vi "Untitled 13 (SubVI)original.vi"(0 "time":dbl[](array[numeric]), 5 "acceleration":dbl[](array[numeric])) -> (1 "Frequency Interval: delta(f)":dbl, 2 "Spectrum plot":cluster{i32, dbl, "spectrum out":dbl[]}(graph), 3 "size(s)":i32, 4 "all rows":dbl[](array[numeric]), 6 "df (Hz)":dbl, 8 "Array":dbl[](array[numeric]), 10 "xf (frequency)":dbl[](array[numeric]), 12 "ploted signal from each selected frequency":dbl[][](graph), 14 "phase 2":dbl[](array[numeric]), 15 "magnitude 2":dbl[](array[numeric]))   [LabVIEW 2020]
uses:
  <vilib>/Analysis/2dsp.llb/Real FFT.vi
  <vilib>/Analysis/NI_AALPro.lvlib
  <vilib>/rvi/Analysis/host/Public/NI_FpgaMspHost.lvlib
  <vilib>/ptbypt/NI_PtbyPt.lvlib
panel:
  out "XY Graph":cluster{dbl[], dbl[]}(graph)
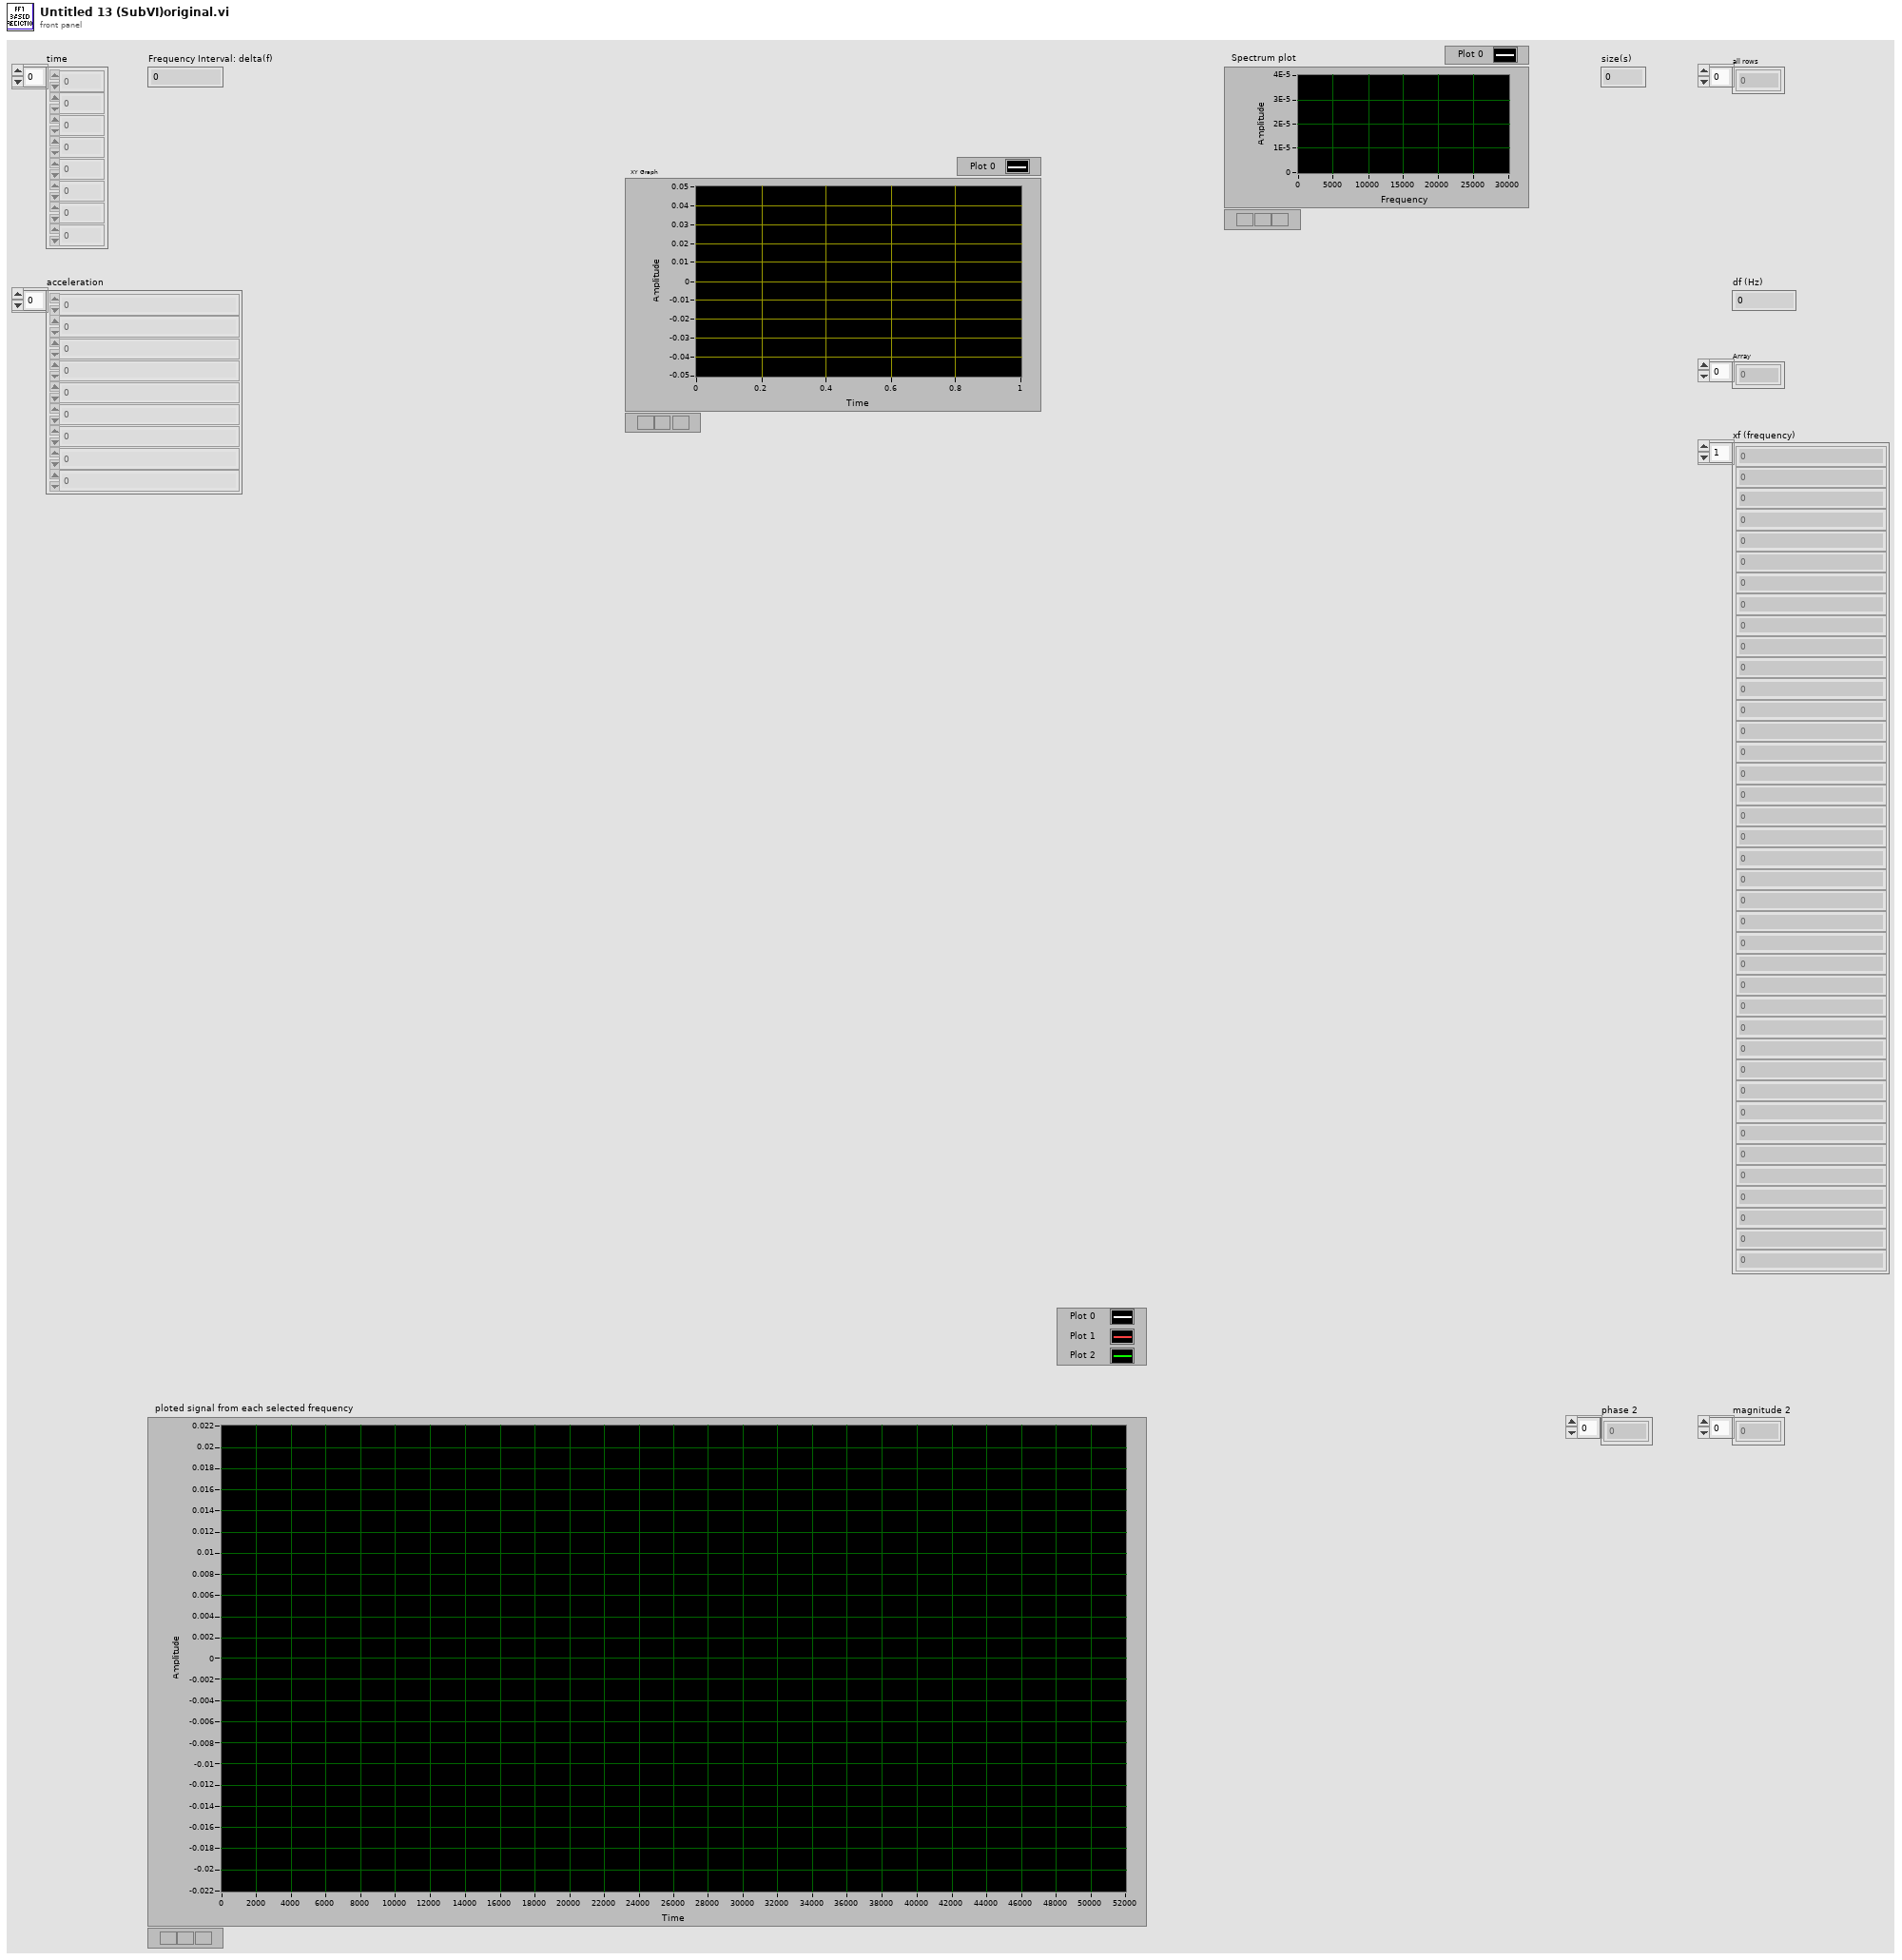
[diagram p1: front panel]
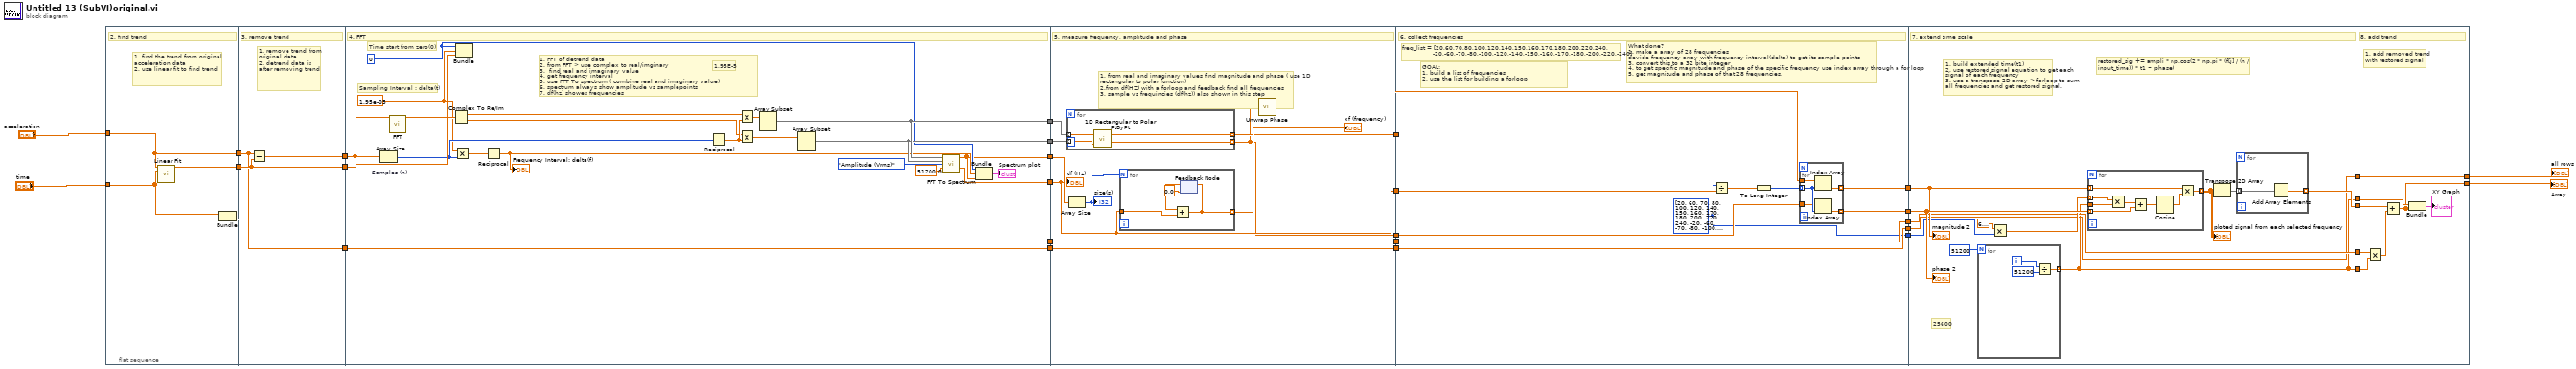
[diagram p0: block diagram]
diagram:
  n1 = flat-sequence {
    tunnel: [w33] -> w30
    tunnel: [w32] -> w29
    tunnel: "acceleration" -> [w32]
    tunnel: "time" -> [w31]
    tunnel: w30 -> [w35]
    tunnel: w29 -> [w34]
    tunnel: [w36] -> w28
    tunnel: [w35] -> w27
    tunnel: [w34] -> w26
    tunnel: w28 -> [w51]
    tunnel: [w50] -> w25
    tunnel: [w49] -> w24
    tunnel: [w42] -> w23
    tunnel: [w38] -> w22
    tunnel: [w37] -> w21
    tunnel: w27 -> [w37]
    tunnel: w26 -> [w40]
    tunnel: [w40] -> w20
    tunnel: w25 -> [w67]
    tunnel: w24 -> [w66]
    tunnel: w23 -> [w62]
    tunnel: w22 -> [w64]
    tunnel: [w62] -> w19
    tunnel: [w61] -> w18
    tunnel: [w60] -> w17
    tunnel: [w59] -> w16
    tunnel: w21 -> [w59]
    tunnel: w20 -> [w58]
    tunnel: [w58] -> w15
    tunnel: w19 -> [w77]
    tunnel: [w83] -> w14
    tunnel: w18 -> [w82]
    tunnel: w17 -> [w81]
    tunnel: [w80] -> w13
    tunnel: [w76] -> w12
    tunnel: [w79] -> w11
    tunnel: w16 -> [w79]
    tunnel: w15 -> [w78]
    tunnel: [w78] -> w10
    tunnel: w14 -> [w100]
    tunnel: w13 -> [w101]
    tunnel: w12 -> [w96]
    tunnel: [w94] -> w9
    tunnel: [w93] -> w8
    tunnel: w11 -> [w93]
    tunnel: [w92] -> w7
    tunnel: [w92] -> w6
    tunnel: w10 -> [w91]
    tunnel: [w91] -> w5
    tunnel: w9 -> [w123]
    tunnel: w8 -> [w121]
    tunnel: w7 -> [w122]
    tunnel: w6 -> [w120]
    tunnel: [w119] -> w2
    tunnel: w5 -> [w119]
    tunnel: [w118] -> w3
    frame #0 {
      # "1. find the trend from original acceleration data\n2. use linear fit to find trend"
      # "2. find trend"
      n2 = call <vilib>:"Linear Fit.vi"("Y"=w32, "X"=w31) -> ("Best Linear Fit"=w33:dbl[])  [unwired: 9 in, 4 out]
      n3 = Bundle("time"=w31, "Best Linear Fit"=w33) -> ()  [unwired: 1 in, 1 out]
    }
    frame #1 {
      # "1. remove trend from original data\n2. detrend data is after removing trend"
      # "3. remove trend"
      n4 = Subtract(x=w34, y=w35) -> (x-y=w36:dbl[])
    }
    frame #2 {
      w39 = 1.95e-05
      w47 = 0
      # "1.95E-5"
      # "1. FFT of detrend data\n2. from FFT > use complex to real/imginary\n3.  find real and imaginary value\n4. get frequency interval\n5. use FFT To spectrum ( combine real and imaginary value)\n6. spectrum always show amplitude vs samplepoints\n7. df(hz) showes frequencies"
      # "Sampling Interval : delta(t)"
      # "Time start from zero(0)"
      # "4. FFT"
      n5 = Array Size "Samples (n)"(array=w51) -> (size(s)=w43:i32)
      n6 = call-poly <vilib>:"FFT.vi"("X"=w51) -> ("FFT {X}"=w45:cdb[])  [unwired: 9 in, 1 out]
      n7 = Complex To Re/Im(x + iy=w45) -> (x=w56:dbl[], y=w55:dbl[])
      n8 = Multiply(x=w39, y=w43) -> (x*y=w52:dbl)
      n9 = Bundle(w47, w39, w51) -> ()  [unwired: 1 in, 1 out]
      n10 = Reciprocal(x=w52) -> (1/x=w44:dbl)
      "Frequency Interval: delta(f)" <- w44
      n11 = Reciprocal(x=w43) -> (1/x=w57:dbl)
      n12 = Multiply(x=w56, y=w57) -> (x*y=w53:dbl[])
      n13 = Multiply(x=w55, y=w57) -> (x*y=w54:dbl[])
      n14 = Array Subset(array=w53) -> (w50:dbl[])  [unwired: 2 in]
      n15 = Array Subset(array=w54) -> (w49:dbl[])  [unwired: 2 in]
      n16 = call <vilib>:"FFT To Spectrum.vi"("real FFT data"=w50, "imaginary FFT data"=w49, "spectrum type"=enum8{"Power (Vrms^2)", "Amplitude (Vrms)"}."Amplitude (Vrms)", "sample rate (S/s)"=51200.0) -> ("spectrum out"=w38:dbl[], "df (Hz)"=w42:dbl)  [unwired: 9 in, 1 out]
      n17 = Bundle(w47, w44, "spectrum out"=w38) -> (→"Spectrum plot":cluster{i32, dbl, "spectrum out":dbl[]})  [unwired: 1 in]
    }
    frame #3 {
      # "1. from real and imaginary values find magnitude and phase ( use 1D rectangular to polar function)\n2.from df(HZ) with a forloop and feedback find all frequencies \n3. sample vs frequincies (df(hz)) also shown in this step"
      # "5. measure frequency, amplitude and phase"
      n18 = for {
        tunnel: w67 -> [w75] mode=indexing
        tunnel: w66 -> [w74] mode=indexing
        tunnel: [w72] -> w61 mode=indexing
        tunnel: [w73] -> w60 mode=indexing
        n19 = call <vilib>:"1D Rectangular to Polar PtByPt.vi"("y"=w74, "x"=w75) -> ("phase"=w73:dbl, "magnitude"=w72:dbl)
      }
      n20 = Array Size(array=w64) -> (size(s)=w65:i32)
      "size(s)" <- w65
      n21 = for {
        N: w65 -> [_]
        tunnel: w62 -> [w70]
        tunnel: [w68] -> w63 mode=indexing
        n22 = feedback #1(0.0) -> (w71:dbl)
        n23 = Add(x=w71, y=w70) -> (x+y=w68:dbl)
        n24 = feedback-in #1(w68) -> ()
      }
      "xf (frequency)" <- w63
      n25 = call <vilib>:"Unwrap Phase.vi"("Phase"=w60) -> ()  [unwired: 9 in, 2 out]
      "df (Hz)" <- w62
    }
    frame #4 {
      w76 = i32[] [20, 60, 70, 80, 100, 120, 140, 150, 160, 170, 180, 200, 220, 240, -20, -60, -70, -80, -100, -120, -140, -150, -160, -170, -180, -200, -220]
      # "What done?\n1. make a array of 28 frequencies\ndevide frequency array with frequency interval(delta) to get its sample points\n3. convert this to a 32 bite integer\n4. to get specific magnitude and phase of the specific frequency use index array through a for loop\n5. get magnitude and phase of that 28 frequencies."
      # "freq_list = [20,60,70,80,100,120,140,150,160,170,180,200,220,240,\n                -20,-60,-70,-80,-100,-120,-140,-150,-160,-170,-180,-200,-220,-240]"
      # "GOAL:\n1. build a list of frequencies\n2. use the list for building a forloop"
      # "6. collect frequencies"
      n26 = Divide(x=w76, y=w77) -> (x/y=w85:dbl[])
      n27 = To Long Integer(number=w85) -> (32bit integer=w84:i32[])
      n28 = for {
        tunnel: w84 -> [w88] mode=indexing
        tunnel: w82 -> [w90]
        tunnel: [w89] -> w83 mode=indexing
        tunnel: w81 -> [w87]
        tunnel: [w86] -> w80 mode=indexing
        n29 = Index Array(array=w90, index=w88) -> (element=w89:dbl)
        n30 = Index Array(array=w87, index=w88) -> (element=w86:dbl)
      }
    }
    frame #5 {
      # "25600"
      # "1. build extended time(t1)\n2. use restored signal equation to get each signal of each frequency\n3. use a transpose 2D array > forloop to sum all frequencies and get restored signal."
      # "restored_sig += ampli * np.cos(2 * np.pi * (f[j] / (n / input_time)) * t1 + phase)"
      # "7. extend time scale"
      n31 = for {
        N: 51200 -> [_]
        tunnel: [w105] -> w92 mode=indexing
        i -> [w107]
        n32 = Divide(x=w107, y=51200) -> (x/y=w105:dbl)
      }
      n33 = Multiply(x=6.283185307179586, y=w96) -> (x*y=w95:dbl[])
      n34 = for {
        tunnel: w92 -> [w115]
        tunnel: w101 -> [w113] mode=indexing
        tunnel: w100 -> [w112] mode=indexing
        tunnel: [w111] -> w99 mode=indexing
        tunnel: w95 -> [w110] mode=indexing
        n35 = Multiply(x=w110, y=w115) -> (x*y=w114:dbl[])
        n36 = Add(x=w114, y=w113) -> (x+y=w109:dbl[])
        n37 = Cosine(x=w109) -> (cos(x)=w108:dbl[])
        n38 = Multiply(x=w112, y=w108) -> (x*y=w111:dbl[])
      }
      "ploted signal from each selected frequency" <- w99
      n39 = Transpose 2D Array(2D array=w99) -> (transposed array=w98:dbl[][])
      n40 = for {
        tunnel: w98 -> [w104] mode=indexing
        tunnel: [w103] -> w94 mode=indexing
        n41 = Add Array Elements(numeric array=w104) -> (sum=w103:dbl)
      }
      "magnitude 2" <- w100
      "phase 2" <- w101
    }
    frame #6 {
      # "1. add removed trend with restored signal"
      # "8. add trend"
      n42 = Multiply(x=w121, y=w120) -> (x*y=w116:dbl[])
      n43 = Add(x=w123, y=w116) -> (x+y=w118:dbl[])
      n44 = Bundle(w122, w118) -> (→"XY Graph":cluster{dbl[], dbl[]})  [unwired: 1 in]
    }
  }
  "all rows" <- w2
  "Array" <- w3
